vi "SeeInvitation.vi"(11 "DataIn":T1) -> (3 "DataOut":T1)   [LabVIEW 2017]
doc: "SubVI criada para mostrar tela de convite a usuário"
uses:
  controls/DataIn.ctl
  controls/Tabuleiro.ctl
  controls/GameOption.ctl
  controls/Table.ctl
  <vilib>/Utility/file.llb/Write Delimited Spreadsheet (string).vi
  <vilib>/Utility/file.llb/Read Delimited Spreadsheet (string).vi
panel:
  out "Convite":string
  in  "Recusar":bool
  in  "Aceitar":bool
  # "Convite!"
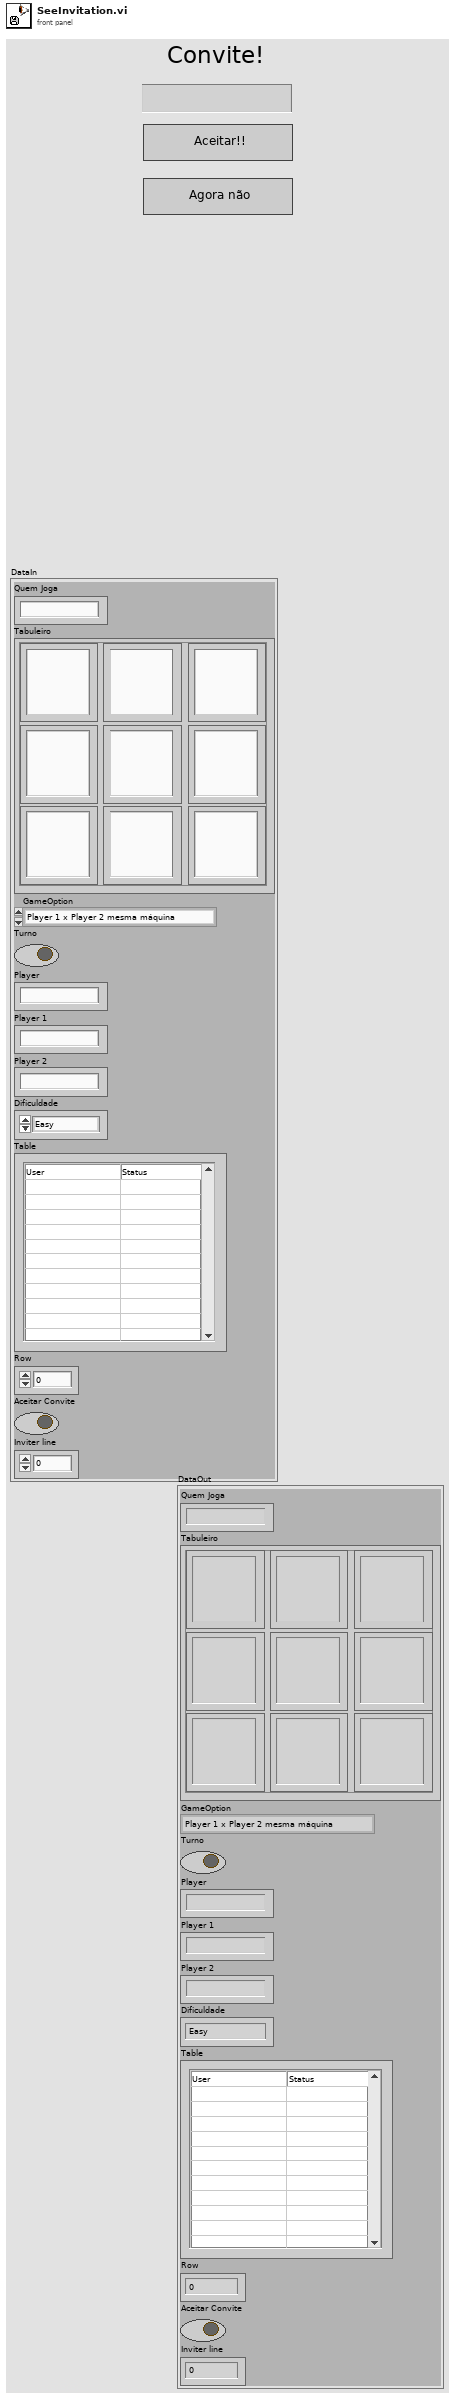
[diagram p1: front panel]
types:
  T1 = typedef "DataIn.ctl" = cluster{"Quem Joga":string, "Tabuleiro":T2, "GameOption":T3, "Turno":bool, "Player":string, "Player 1":string, "Player 2":string, "Dificuldade":enum16{"Easy", "Medium", "Hard"}, "Table":T4, "Row":u32, "Aceitar Convite":bool, "Inviter line":u32}
  T2 = typedef "Tabuleiro.ctl" = cluster{"(0,0)":string, "(1,0)":string, "(0,1)":string, "(1,1)":string, "(2,0)":string, "(1,2)":string, "(2,2)":string, "(0,2)":string, "(2,1) ":string}
  T3 = typedef "GameOption.ctl" = enum16{"Player 1 x Player 2 mesma máquina", "Player 1 x Player 2 pela rede", "Player 1 x Computador", "Wait for Event", "Initialize", "Stop"}
  T4 = typedef "Table.ctl" = string[][]
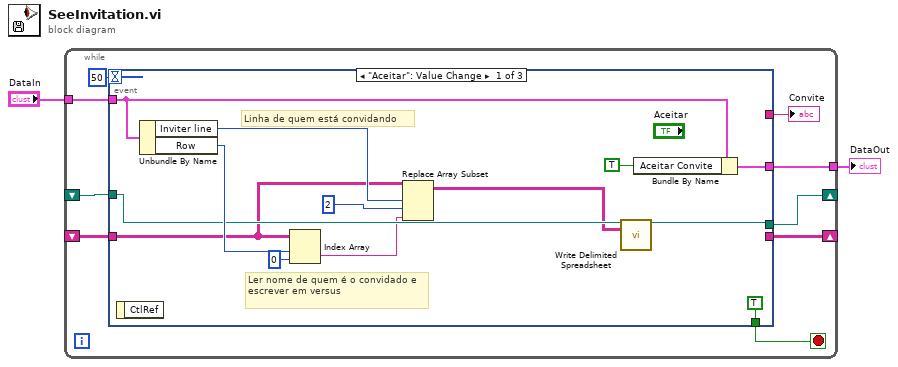
[diagram p0: block diagram]
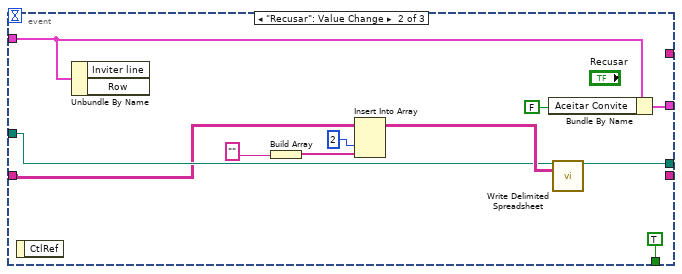
[diagram p2: hidden frame]
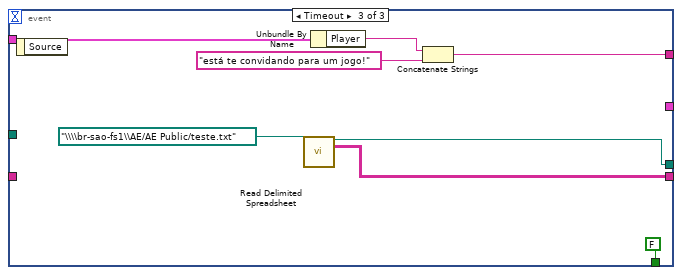
[diagram p3: hidden frame]
diagram:
  n1 = while {
    tunnel: "DataIn" -> [w11]
    tunnel: [w10] -> w1
    shift-right: [w6] -> _
    shift-left: _ -> [w5]
    shift-right: [w4] -> _
    shift-left: _ -> [w3]
    stop <- w8 stop-if-true
    n2 = event shown="[0] \"Aceitar\": Value Change" {
      selector: _ -> [_ _ _]
      dyn-events: _ -> [_ _ _]
      timeout: 50 -> [_ _ _]
      tunnel: [w24 w35 _] -> w10
      tunnel: w11 -> [w12 w30 w41]
      tunnel: [_ _ w40] -> w7
      tunnel: [TRUE TRUE FALSE] -> w8
      tunnel: [w15 w28 w37] -> w6
      tunnel: w5 -> [w18 w29 _]
      tunnel: [_ _ w36] -> w4
      tunnel: w3 -> [w16 w27 _]
      event "Aceitar": Value Change {
        # "Ler nome de quem é o convidado e escrever em versus"
        # "Linha de quem está convidando"
        n3 = event-data() -> ()  [unwired: 1 in, 1 out]
        n4 = Unbundle By Name(w12) -> ("Inviter line"=w21:u32, "Row"=w20:u32)
        n5 = Index Array(array=w16, index (row)=w20, index (col)=0 ("disabled index (col)")) -> (element=w13:string)
        n6 = Replace Array Subset(array=w16, new element=w13, index (row)=w21, index (col)=2 ("disabled index (col)")) -> (w17:string[][])
        n7 = call-poly <vilib>:"Write Delimited Spreadsheet.vi"("file path (dialog if empty)"=w18, "2D data"=w17) -> ("new file path (Not A Path if cancelled)"=w15:path)  [unwired: 12 in, 1 out]
        n8 = Bundle By Name(cluster=w12, "Aceitar Convite"=TRUE) -> (w24:T1)
      }
      event "Recusar": Value Change {
        n9 = event-data() -> ()  [unwired: 1 in, 1 out]
        n10 = Unbundle By Name(w30) -> ()  [unwired: 2 out]
        n11 = Build Array("") -> (w25:string[])
        n12 = Insert Into Array(array=w27, index (col)=2 ("disabled index (col)"), new element=w25) -> (w32:string[][])  [unwired: 1 in]
        n13 = Bundle By Name(cluster=w30, "Aceitar Convite"=FALSE) -> (w35:T1)
        n14 = call-poly <vilib>:"Write Delimited Spreadsheet.vi"("file path (dialog if empty)"=w29, "2D data"=w32) -> ("new file path (Not A Path if cancelled)"=w28:path)  [unwired: 12 in, 1 out]
      }
      event Timeout {
        n15 = event-data() -> ()  [unwired: 1 in, 1 out]
        n16 = call-poly <vilib>:"Read Delimited Spreadsheet.vi"("file path (dialog if empty)"=path "\\\\br-sao-fs1\\AE/AE Public/teste.txt" ("file path (use dialog)")) -> ("new file path (Not A Path if cancelled)"=w37:path, "all rows"=w36:string[][])  [unwired: 9 in, 4 out]
        n17 = Unbundle By Name(w41) -> ("Player"=w43:string)
        n18 = Concatenate Strings(w43, "está te convidando para um jogo!" ("string")) -> (w40:string)
      }
    }
    "Convite" <- w7
  }
  "DataOut" <- w1
